vi "TargetAndLoad.vi"   [LabVIEW 2015]
uses:
  MotorPositionGlobals.vi
  GlobalVisionVars.vi
  VisionGlobals.vi
types:
  T1 = typedef "WPI_DigitalOutputDevRef.ctl" = cluster{"DIO Channel":T2, "DevStatus":errorcluster}
  T2 = typedef "FPGA_DIOChannel.ctl" = enum8{"DIO 0", "DIO 1", "DIO 2", "DIO 3", "DIO 4", "DIO 5", "DIO 6", "DIO 7", "DIO 8", "DIO 9", "DIO MXP 0", "DIO MXP 1", "DIO MXP 2", "DIO MXP 3", "DIO MXP 4", "DIO MXP 5", "DIO MXP 6", "DIO MXP 7", "DIO MXP 8", "DIO MXP 9", "DIO MXP 10", "DIO MXP 11", "DIO MXP 12", "DIO MXP 13", "DIO MXP 14", "DIO MXP 15", "Invalid"}
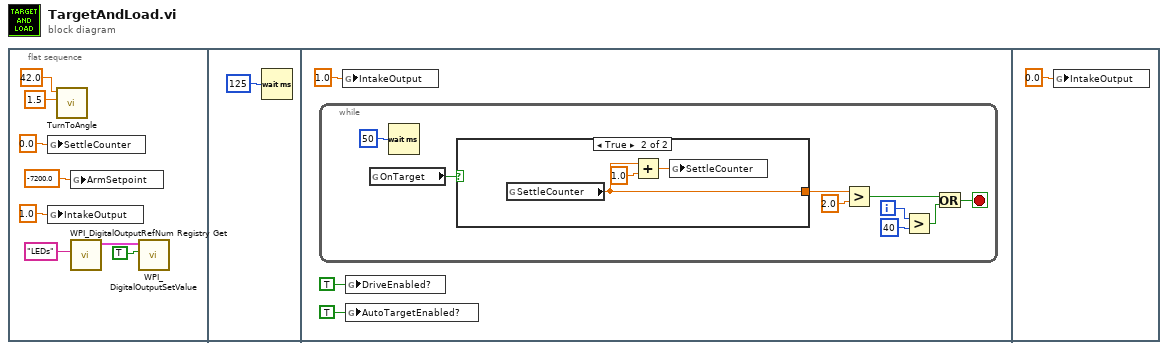
[diagram p0: block diagram]
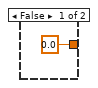
[diagram p2: hidden frame]
diagram:
  n1 = flat-sequence {
    frame #0 {
      n2 = global write "GlobalVisionVars.vi" "SettleCounter"(0.0 ("SettleCounter")) -> ()
      n3 = global write "MotorPositionGlobals.vi" "IntakeOutput"(1.0 ("IntakeOutput")) -> ()
      n4 = call "TurnToAngle.vi"("AllowedDeviation"=1.5, "GyroValue"=42.0) -> ()  [unwired: 10 in]
      n5 = global write "MotorPositionGlobals.vi" "ArmSetpoint"(-7200.0 ("ArmSetpoint")) -> ()
      n6 = call <vilib>:"WPI_DigitalOutputRefNum Registry Get.vi"("refnum name"="LEDs") -> ("DigitalOutputDevRef"=w4:T1)  [unwired: 9 in, 1 out]
      n7 = call <vilib>:"WPI_DigitalOutputSetValue.vi"("Value"=TRUE, "DigitalOutputDevRef"=w4) -> ()  [unwired: 8 in, 2 out]
    }
    frame #1 {
      n8 = Wait (ms)(milliseconds to wait=u32 125) -> ()  [unwired: 1 out]
    }
    frame #2 {
      n9 = while {
        i -> [w19]
        stop <- w20 stop-if-true
        n10 = global read "GlobalVisionVars.vi" "OnTarget"() -> (w16:bool)
        n11 = Wait (ms)(milliseconds to wait=u32 50) -> ()  [unwired: 1 out]
        n12 = case shown="True" w16 {
          tunnel: [0.0 ("SettleCounter") w23] -> w13
          frame False {
          }
          frame True {
            n13 = global read "GlobalVisionVars.vi" "SettleCounter"() -> (w23:dbl)
            n14 = Add(x=w23, y=1.0) -> (x+y=w24:dbl)
            n15 = global write "GlobalVisionVars.vi" "SettleCounter"(w24) -> ()
          }
        }
        n16 = Greater?(x=w13, y=2.0) -> (0:w14:bool)
        n17 = Greater?(x=w19, y=40) -> (0:w17:bool)
        n18 = Or(x=w14, y=w17) -> (x .or. y?=w20:bool)
      }
      n19 = global write "MotorPositionGlobals.vi" "IntakeOutput"(1.0 ("IntakeOutput")) -> ()
      n20 = global write "VisionGlobals.vi" "DriveEnabled?"(TRUE ("DriveEnabled?")) -> ()
      n21 = global write "VisionGlobals.vi" "AutoTargetEnabled?"(TRUE ("AutoTargetEnabled?")) -> ()
    }
    frame #3 {
      n22 = global write "MotorPositionGlobals.vi" "IntakeOutput"(0.0 ("IntakeOutput")) -> ()
    }
  }
